vi "AB_CheckMultibyte.vi"(8 "error in (no error)":errorcluster, 11 "generated files":path[](array[path])) -> (0 "error out":errorcluster, 3 "generated files out":path[](array[path]))   [LabVIEW 2020]
uses:
  <resource>/Framework/Providers/Common/provcom_StringGlobals.vi
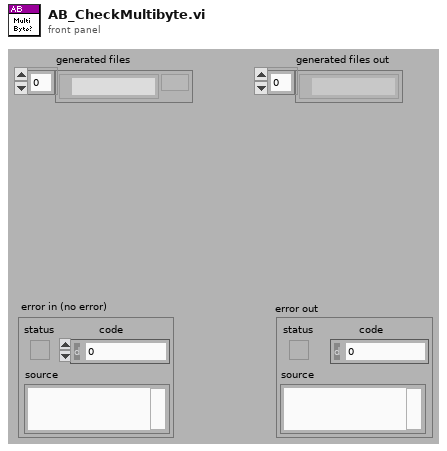
[diagram p1: front panel]
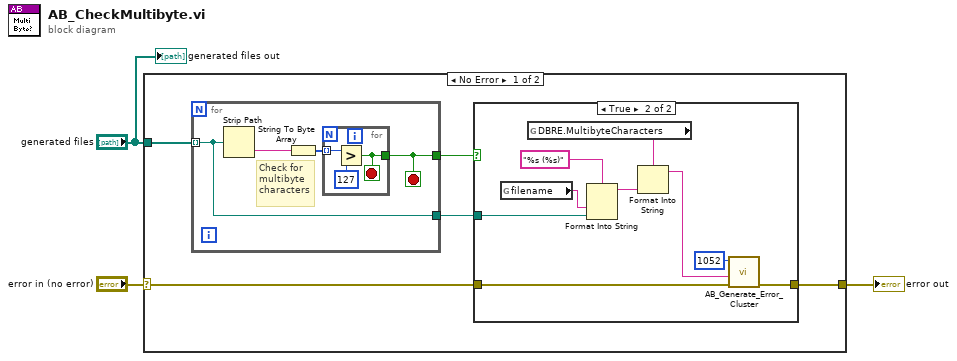
[diagram p0: block diagram]
diagram:
  n1 = case shown="No Error" "error in (no error)" {
    selector: "error in (no error)" -> [w5 w26]
    tunnel: [w4 w26] -> w3
    tunnel: "generated files" -> [w8 _]
    frame No Error {
      n2 = for {
        tunnel: w8 -> [w20] mode=indexing
        tunnel: [w20] -> w6
        tunnel: [w21] -> w7
        stop <- w21 stop-if-true
        # "Check for\nmultibyte\ncharacters"
        n3 = Strip Path(path=w20) -> (name=w19:string)  [unwired: 1 out]
        n4 = String To Byte Array(string=w19) -> (unsigned byte array=w22:u8[])
        n5 = for {
          tunnel: w22 -> [w25] mode=indexing
          tunnel: [w23] -> w21
          stop <- w23 stop-if-true
          n6 = Greater?(x=w25, y=u8 127) -> (0:w23:bool)
        }
      }
      n7 = case shown="True" w7 {
        tunnel: w6 -> [_ w13]
        tunnel: w5 -> [w9 w12]
        tunnel: [w9 w11] -> w4
        frame False {
        }
        frame True {
          n8 = global read "provcom_StringGlobals.vi" "filename"() -> (w16:string)
          n9 = global read "provcom_StringGlobals.vi" "DBRE.MultibyteCharacters"() -> (w10:string)
          n10 = Format Into String(format string="%s (%s)", w16, w13) -> (resulting string=w17:string)  [unwired: 2 in, 1 out]
          n11 = Format Into String(format string=w10, w17) -> (resulting string=w18:string)  [unwired: 2 in, 1 out]
          n12 = call <vilib>:"AB_Generate_Error_Cluster.vi"("error in (no error)"=w12, "Additional Message"=w18, "Code"=1052) -> ("error out"=w11:errorcluster)  [unwired: 1 in, 7 out]
        }
      }
    }
    frame Error {
    }
  }
  "error out" <- w3
  "generated files out" <- "generated files"
